vi "water sound.vi"(10 "Path 2":path, 11 "Path":path) -> ()   [LabVIEW 2013]
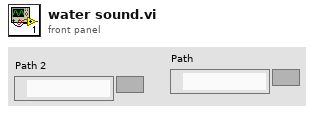
[diagram p1: front panel]
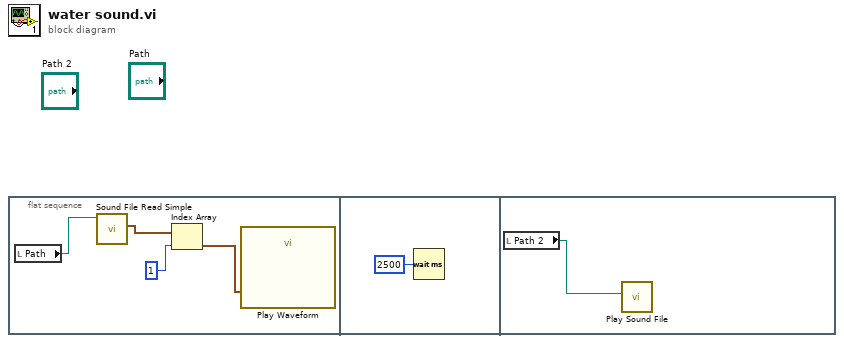
[diagram p0: block diagram]
diagram:
  n1 = flat-sequence {
    frame #0 {
      n2 = local read "Path"() -> (w4:path)
      n3 = call <vilib>:"Sound File Read Simple.vi"("path"=w4) -> ("data"=w3:waveform(dbl)[])  [unwired: 7 in, 3 out]
      n4 = Index Array(array=w3, index=1) -> (element=w1:waveform(dbl))
      n5 = call "Play Waveform"("Data"=w1) -> ()  [unwired: 18 in, 1 out]
    }
    frame #1 {
      n6 = Wait (ms)(milliseconds to wait=u32 2500) -> ()  [unwired: 1 out]
    }
    frame #2 {
      n7 = local read "Path 2"() -> (w6:path)
      n8 = call <vilib>:"Play Sound File.vi"("path"=w6) -> ()  [unwired: 9 in, 2 out]
    }
  }
